vi "Test Stack Preview Elements.vi"() -> ()   [LabVIEW 2013]
uses:
  Circular Buffers/VariantBuffer/buffer-type -- enum.ctl
  <vilib>/addons/_JKI Toolkits/Caraya/classes/Assert/Assert True.vi
  Circular Buffers/VariantBuffer/VariantBuffer.lvclass
  <vilib>/addons/_JKI Toolkits/Caraya/classes/Assert/Assert.lvclass
  <vilib>/addons/_JKI Toolkits/Caraya/classes/Test/Test.lvclass
panel:
  out "elements 7":variant[](array[variant])
  out "elements 6":variant[](array[variant])
  out "elements 5":variant[](array[variant])
  out "elements 4":variant[](array[variant])
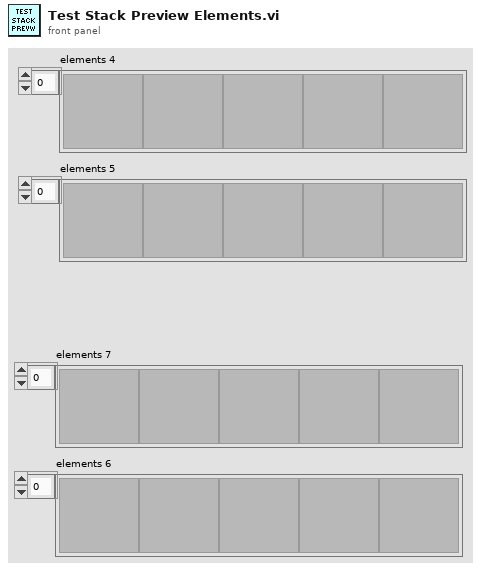
[diagram p1: front panel]
types:
  T1 = typedef "CircularBuffer.lvlib/VariantBuffer.lvclass/buffer-type -- enum.ctl" = enum16{"Queue", "Stack"}
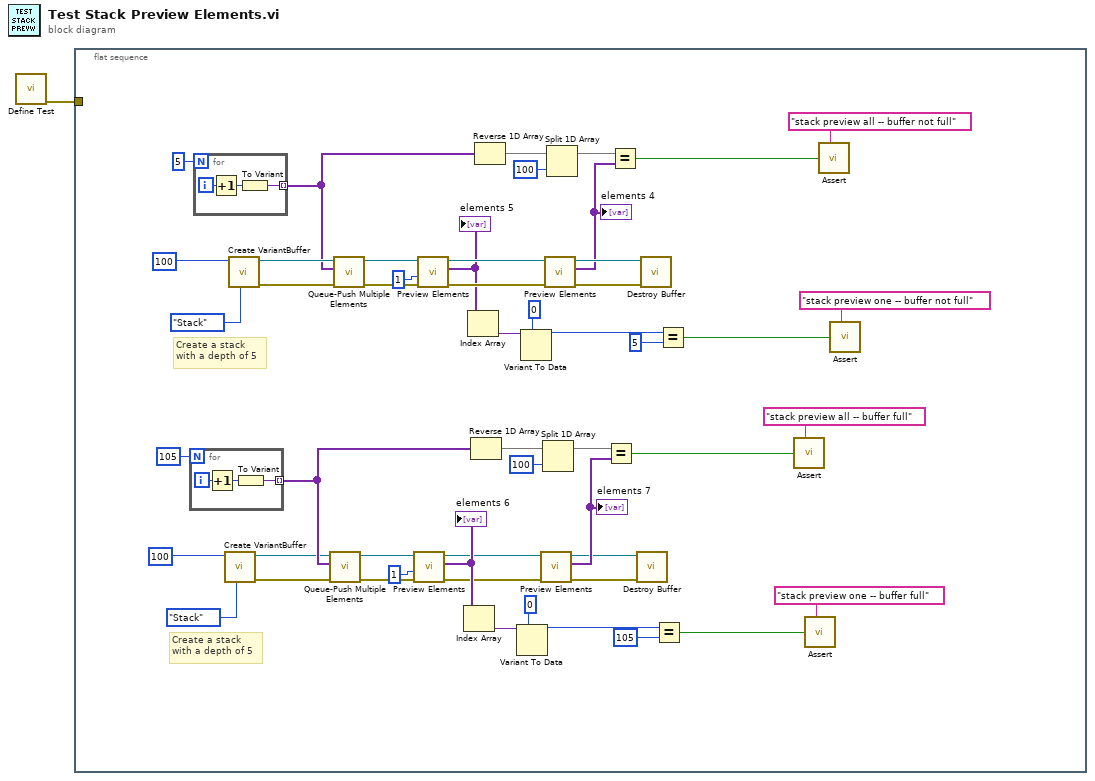
[diagram p0: block diagram]
diagram:
  n1 = call <vilib>:"Define Test.vi"() -> ("error out"=w1:errorcluster)  [unwired: 10 in, 1 out]
  n2 = flat-sequence {
    tunnel: w1 -> [_]
    frame #0 {
      # "Create a stack\nwith a depth of 5"
      # "Create a stack\nwith a depth of 5"
      n3 = for {
        N: 105 -> [_]
        tunnel: [w55] -> w19 mode=indexing
        i -> [w56]
        n4 = Increment(x=w56) -> (x+1=w54:i32)
        n5 = To Variant(anything=w54) -> (Variant=w55:variant)
      }
      n6 = for {
        N: 5 -> [_]
        tunnel: [w58] -> w40 mode=indexing
        i -> [w59]
        n7 = Increment(x=w59) -> (x+1=w57:i32)
        n8 = To Variant(anything=w57) -> (Variant=w58:variant)
      }
      n9 = call "Create VariantBuffer.vi"("buffer-type"=buffer-type_--_enum."Stack", "bufSize"=100) -> ("error out"=w10:errorcluster, "Buffer"=w9:refnum<data-value>)  [unwired: 8 in]
      n10 = call "Create VariantBuffer.vi"("buffer-type"=buffer-type_--_enum."Stack", "bufSize"=100) -> ("error out"=w49:errorcluster, "Buffer"=w50:refnum<data-value>)  [unwired: 8 in]
      n11 = call "Queue-Push Multiple Elements.vi"("error in"=w10, "elements"=w19, "Buffer in"=w9) -> ("error out"=w16:errorcluster, "Buffer"=w14:refnum<data-value>)  [unwired: 6 in, 1 out]
      n12 = call "Queue-Push Multiple Elements.vi"("error in"=w49, "elements"=w40, "Buffer in"=w50) -> ("error out"=w43:errorcluster, "Buffer"=w45:refnum<data-value>)  [unwired: 6 in, 1 out]
      n13 = call "Preview Elements.vi"("error in"=w16, "count (-1: all)"=1, "ByteBuffer in"=w14) -> ("error out"=w17:errorcluster, "elements"=w26:variant[], "ByteBuffer"=w15:refnum<data-value>)  [unwired: 6 in]
      "elements 6" <- w26
      n14 = call "Preview Elements.vi"("error in"=w43, "count (-1: all)"=1, "ByteBuffer in"=w45) -> ("error out"=w42:errorcluster, "elements"=w33:variant[], "ByteBuffer"=w44:refnum<data-value>)  [unwired: 6 in]
      "elements 5" <- w33
      n15 = Index Array(array=w26) -> (element=w22:variant)  [unwired: 1 in]
      n16 = Index Array(array=w33) -> (element=w37:variant)  [unwired: 1 in]
      n17 = Reverse 1D Array(array=w19) -> (reversed array=w28:variant[])
      n18 = Reverse 1D Array(array=w40) -> (reversed array=w31:variant[])
      n19 = Variant To Data(type=0 ("count (-1: all)"), Variant=w22) -> (data=w23:i32)  [unwired: 1 in, 1 out]
      n20 = Variant To Data(type=0 ("count (-1: all)"), Variant=w37) -> (data=w36:i32)  [unwired: 1 in, 1 out]
      n21 = call "Preview Elements.vi"("error in"=w17, "ByteBuffer in"=w15) -> ("error out"=w12:errorcluster, "elements"=w18:variant[], "ByteBuffer"=w11:refnum<data-value>)  [unwired: 7 in]
      "elements 7" <- w18
      n22 = Split 1D Array(array=w28, index=100) -> (first subarray=w29:variant[])  [unwired: 1 out]
      n23 = call "Preview Elements.vi"("error in"=w42, "ByteBuffer in"=w44) -> ("error out"=w47:errorcluster, "elements"=w41:variant[], "ByteBuffer"=w48:refnum<data-value>)  [unwired: 7 in]
      "elements 4" <- w41
      n24 = Split 1D Array(array=w31, index=100) -> (first subarray=w30:variant[])  [unwired: 1 out]
      n25 = Equal?(x=w29, y=w18) -> (x = y?=w20:bool)
      n26 = Equal?(x=w30, y=w41) -> (x = y?=w39:bool)
      n27 = call "Destroy Buffer.vi"("error in"=w12, "Buffer"=w11) -> ()  [unwired: 8 in, 2 out]
      n28 = call "Destroy Buffer.vi"("error in"=w47, "Buffer"=w48) -> ()  [unwired: 8 in, 2 out]
      n29 = Equal?(x=w23, y=105 ("count (-1: all)")) -> (x = y?=w25:bool)
      n30 = Equal?(x=w36, y=5 ("count (-1: all)")) -> (x = y?=w34:bool)
      n31 = call-poly <vilib>:"Assert.vi"("Label"="stack preview all -- buffer full", "True?"=w20) -> ()  [unwired: 8 in, 2 out]
      n32 = call-poly <vilib>:"Assert.vi"("Label"="stack preview one -- buffer full", "True?"=w25) -> ()  [unwired: 8 in, 2 out]
      n33 = call-poly <vilib>:"Assert.vi"("Label"="stack preview all -- buffer not full", "True?"=w39) -> ()  [unwired: 8 in, 2 out]
      n34 = call-poly <vilib>:"Assert.vi"("Label"="stack preview one -- buffer not full", "True?"=w34) -> ()  [unwired: 8 in, 2 out]
    }
  }
